vi "Query Trigger D Source Catalog.vi"(8 "error in (no error)":errorcluster, 10 "Trigger (1)":i32=1, 11 "VISA resource name":refnum<visa-resource-name>) -> (0 "error out":errorcluster, 2 "Sources":string, 3 "VISA resource name out":refnum<visa-resource-name>)   [LabVIEW 2015, in "Rohde&Schwarz CMXP Base.lvlib"]
doc: "Lists all trigger source values that can be set using RSCMXPBASE_ATTR_TRIGGER_D_SOURCE.\n\nAttributes:\nRSCMXPBASE_ATTR_SELECT_TRIGGER\nRSCMXPBASE_ATTR_TRIGGER_D_SOURCE_CATALOG\n\nRemote-control command:\nTRIGger:BASE:EXTD<n>:CATalog:SOURce?"
uses:
  <instrlib>/Rohde&Schwarz CMXP Base/Rohde&Schwarz CMXP Base.lvlib
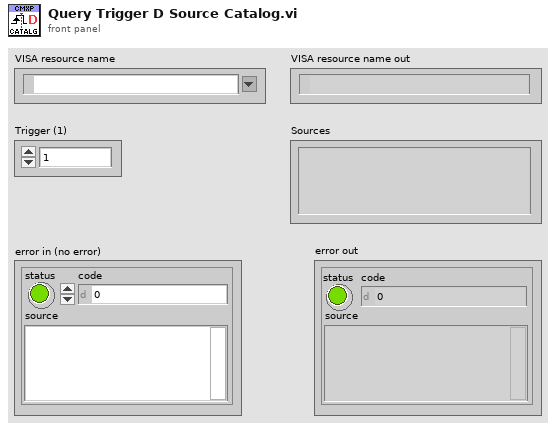
[diagram p1: front panel]
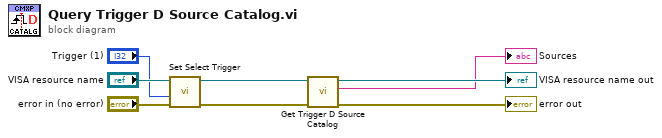
[diagram p0: block diagram]
diagram:
  n1 = call "Set Select Trigger"("error in (no error)"="error in (no error)", "Select Trigger (0)"="Trigger (1)", "instrument handle"="VISA resource name") -> ("error out"=w4:errorcluster, "instrument handle out"=w3:refnum<visa-resource-name>)  [unwired: 7 in]
  n2 = call "Get Trigger D Source Catalog"("error in (no error)"=w4, "instrument handle"=w3) -> ("error out"=→"error out":errorcluster, "Trigger D Source Catalog"=→"Sources":string, "instrument handle out"=→"VISA resource name out":refnum<visa-resource-name>)  [unwired: 7 in]
